vi "DAQmx_Master_or_Slave.vi"(8 "error in (no error)":errorcluster, 11 "DAQmx in":refnum<class "DAQmx.lvclass">) -> (0 "error out":errorcluster, 2 "Enum":enum16{"MASTER", "SLAVE"}(ring), 3 "DAQmx out":refnum<class "DAQmx.lvclass">)   [LabVIEW 2016, in "DAQmx.lvclass"]
uses:
  DAQmx.lvclass
  C:/user/patrick/hg/lockin.SMO/lvsrc/SMOs/DAQ/DAQ.lvclass
  DAQ/Typedefs/DAQType.ctl
  DAQ/Typedefs/PrivateEvents--DAQ.AI.Channels.ctl
  DAQ/DAQ.lvclass/DAQ.ctl
  DAQ/DAQ.lvclass
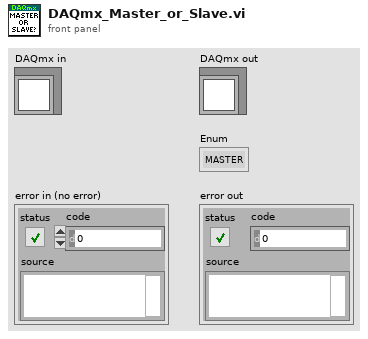
[diagram p1: front panel]
types:
  T1 = typedef "DAQ.lvclass/PrivateEvents--DAQ.AI.Channels.ctl" = string
  T2 = typedef "DAQ.lvclass/DAQType.ctl" = enum16{"AI", "AO"}
  T3 = typedef "DAQ.lvclass/DAQ.Config.ctl" = cluster{"Channels":T1, "DAQType":T2, "minimum value":dbl, "maximum value":dbl, "sampling info":T4, "SamplingMode":T5, "gain":dbl[], "offset":dbl[]}
  T4 = typedef "DAQ.lvclass/SamplingInfo.ctl" = cluster{"Fs":dbl, "#s":dbl}
  T5 = typedef "DAQ.lvclass/SamplingMode.ctl" = enum16{"Continuous", "Finite"}
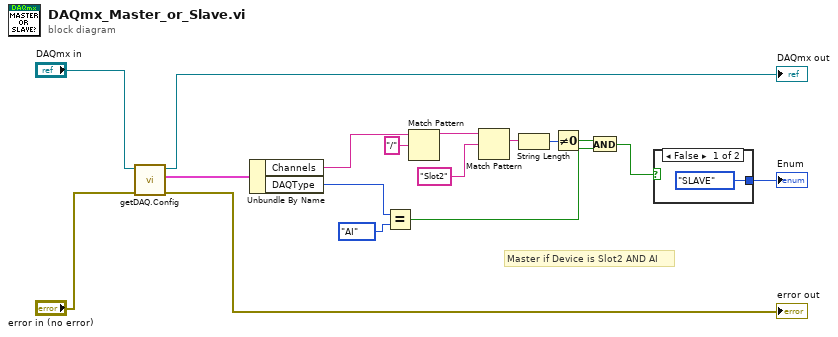
[diagram p0: block diagram]
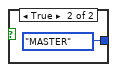
[diagram p2: hidden frame]
diagram:
  # "Master if Device is Slot2 AND AI"
  n1 = call "getDAQ.Config.vi"("error in (no error)"="error in (no error)", "DAQ in"="DAQmx in") -> ("error out"=→"error out":errorcluster, "Configuration"=w15:T3, "DAQ out"=→"DAQmx out":refnum<class "DAQmx.lvclass">)  [unwired: 7 in]
  n2 = Unbundle By Name(w15) -> ("Channels"=w12:T1, "DAQType"=w16:T2)
  n3 = Equal?(x=w16, y=DAQType."AI" ("DAQType")) -> (x = y?=w4:bool)
  n4 = Match Pattern(string=w12, regular expression="/") -> (before substring=w8:T1)  [unwired: 1 in, 3 out]
  n5 = Match Pattern(string=w8, regular expression=T1 "Slot2" ("before substring")) -> (match substring=w7:T1)  [unwired: 1 in, 3 out]
  n6 = String Length(string=w7) -> (length=w6:i32)
  n7 = Not Equal To 0?(x=w6) -> (x != 0?=w5:bool)
  n8 = And(x=w5, y=w4) -> (x .and. y?=w3:bool)
  n9 = case shown="False" w3 {
    tunnel: [enum16{"MASTER", "SLAVE"}."SLAVE" enum16{"MASTER", "SLAVE"}."MASTER"] -> w10
    frame False {
    }
    frame True {
    }
  }
  "Enum" <- w10
